vi "observe_state.vi"(1 "Numeric":u32, 2 "activity":dbl[][](array[numeric])) -> (0 "Cluster":cluster{dbl[], "activity":dbl[]})   [LabVIEW 2009]
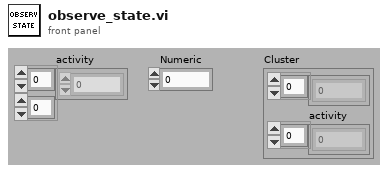
[diagram p1: front panel]
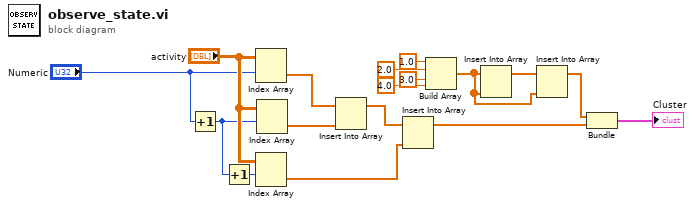
[diagram p0: block diagram]
diagram:
  n1 = Increment(x="Numeric") -> (x+1=w1:u32)
  n2 = Increment(x=w1) -> (x+1=w2:u32)
  n3 = Index Array(array="activity", index (row)="Numeric") -> (element=w3:dbl[])  [unwired: 1 in]
  n4 = Index Array(array="activity", index (row)=w2) -> (element=w6:dbl[])  [unwired: 1 in]
  n5 = Index Array(array="activity", index (row)=w1) -> (element=w4:dbl[])  [unwired: 1 in]
  n6 = Insert Into Array(array=w3, new element=w4) -> (w5:dbl[])  [unwired: 1 in]
  n7 = Insert Into Array(array=w5, new element=w6) -> (w11:dbl[])  [unwired: 1 in]
  n8 = Build Array(1.0 ("element"), 2.0 ("element"), 3.0 ("element"), 4.0 ("element")) -> (w13:dbl[])
  n9 = Insert Into Array(array=w13, new element=w13) -> (w12:dbl[])  [unwired: 1 in]
  n10 = Insert Into Array(array=w12, new element=w13) -> (w15:dbl[])  [unwired: 1 in]
  n11 = Bundle(w15, "activity"=w11) -> (→"Cluster":cluster{dbl[], "activity":dbl[]})  [unwired: 1 in]
